vi "uA_turn_on_off_shunt_bypass.vi"(8 "error in":errorcluster, 10 "USB DAQ":tag="Dev4", 11 "Bypass Shunt":T1(ring)) -> (0 "error out":errorcluster)   [LabVIEW 2015]
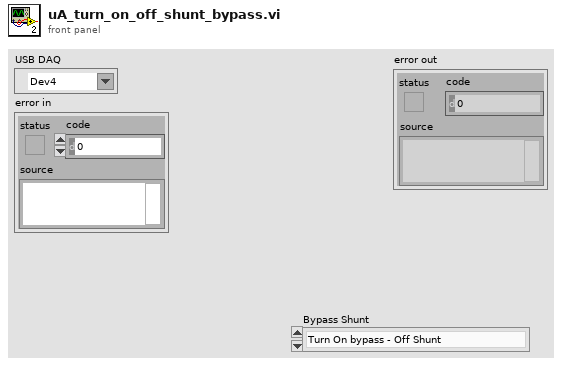
[diagram p1: front panel]
types:
  T1 = enum16{"Turn On bypass - Off Shunt", "Turn Off bypass - On Shunt"}
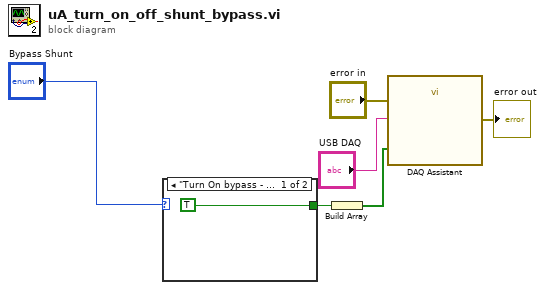
[diagram p0: block diagram]
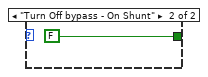
[diagram p2: hidden frame]
diagram:
  n1 = case shown="\"Turn On bypass - Off Shunt\", Default" "Bypass Shunt" {
    tunnel: [TRUE FALSE] -> w5
    frame "Turn On bypass - Off Shunt", Default {
    }
    frame "Turn Off bypass - On Shunt" {
    }
  }
  n2 = Build Array(w5) -> (w4:bool[])
  n3 = call "DAQ Assistant"("data"=w4, "error in"="error in", "device name"="USB DAQ") -> ("error out"=→"error out":errorcluster)  [unwired: 15 in, 1 out]
